vi "LeftOrRight.vi"(10 "Vertex2":T1, 11 "Vertex1":T1) -> (3 "Left/Right":bool)   [LabVIEW 2014]
uses:
  TypeDefs/Point2D.ctl
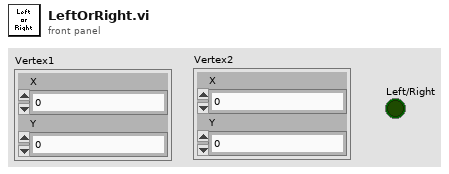
[diagram p1: front panel]
types:
  T1 = typedef "Point2D.ctl" = cluster{"X":sgl, "Y":sgl}
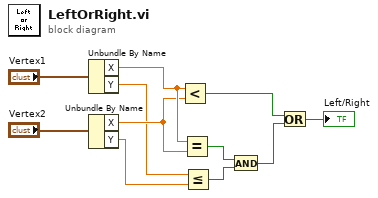
[diagram p0: block diagram]
diagram:
  n1 = Unbundle By Name("Vertex1") -> ("X"=w9:sgl, "Y"=w7:sgl)
  n2 = Unbundle By Name("Vertex2") -> ("X"=w8:sgl, "Y"=w6:sgl)
  n3 = Less?(x=w9, y=w8) -> (x < y?=w3:bool)
  n4 = Equal?(x=w9, y=w8) -> (x = y?=w5:bool)
  n5 = Less Or Equal?(x=w7, y=w6) -> (x <= y?=w4:bool)
  n6 = And(x=w5, y=w4) -> (x .and. y?=w2:bool)
  n7 = Or(x=w3, y=w2) -> (x .or. y?=→"Left/Right":bool)
